vi "ts_tree_set_status.vi"(8 "error in (no error)":errorcluster, 9 "ts.status":bool, 10 "ts.data":T1, 11 "Tree.in":refnum<vi>) -> (0 "error out":errorcluster, 3 "Tree.out":refnum<vi>)   [LabVIEW 2015]
doc: "sets the status symbol (pass/fail glyph) for a given active tag"
uses:
  ts-data.ctl
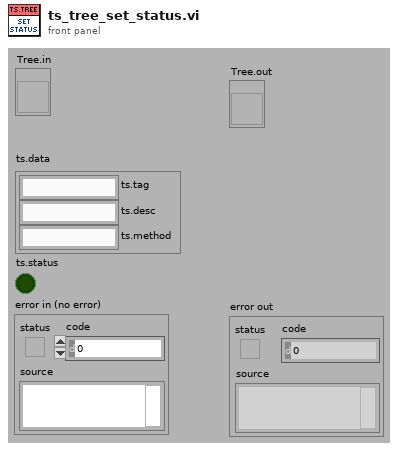
[diagram p1: front panel]
types:
  T1 = typedef "ts-data.ctl" = cluster{"ts.tag":string, "ts.desc":string, "ts.method":string}
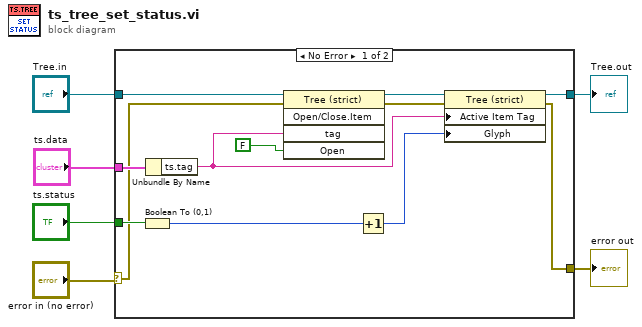
[diagram p0: block diagram]
diagram:
  n1 = case shown="No Error" "error in (no error)" {
    selector: "error in (no error)" -> [w9 w19]
    tunnel: "Tree.in" -> [w11 w20]
    tunnel: [w17 w20] -> w4
    tunnel: [w16 w19] -> w3
    tunnel: "ts.data" -> [w18 _]
    tunnel: "ts.status" -> [w15 _]
    frame No Error {
      n2 = Boolean To (0,1)(Boolean=w15) -> (0, 1=w14:i16)
      n3 = Unbundle By Name(w18) -> ("ts.tag"=w7:string)
      n4 = invoke class="Tree (strict)" method="Open/Close.Item"(reference=w11, error in=w9, "tag"=w7, "Open"=FALSE ("Open?")) -> (reference out=w10:refnum<vi>, error out=w8:errorcluster)  [unwired: 1 in, 3 out]
      n5 = Increment(x=w14) -> (x+1=w13:i16)
      n6 = property class="Tree (strict)"(reference=w10, error in=w8, "Active Item Tag"=w7, "Glyph"=w13) -> (reference out=w17:refnum<vi>, error out=w16:errorcluster)
    }
    frame Error {
    }
  }
  "Tree.out" <- w4
  "error out" <- w3
